vi "Find PID in Configuration.vi"(10 "Channels":T1={"ID"="", "Setpoint"=refnum, "Process Variable"=refnum, "Output"=refnum, "PID gains"={"proportional gain (Kc)"=1.0, "integral time (Ti, min)"=0.01, "derivative time (Td, min)"=0.0}, "output range"={"output high"=100.0, "output low"=-100.0}} {"output range"."output low" format="%.2f"; "output range"."output high" format="%.2f"}, 11 "Tagbus PID Module configuration in":refnum<class "Tagbus PID Module configuration.lvclass">) -> (2 "index":i32, 3 "Tagbus PID Module configuration out":refnum<class "Tagbus PID Module configuration.lvclass">)   [LabVIEW 2014, in "Tagbus PID Module configuration.lvclass"]
doc: "This VI locates a given PID Loop in the Module Configuration and returns it's index if found, or -1 if not found."
uses:
  Tagbus PID Module configuration.lvclass
  <vilib>/NI/Tag Bus Module Framework/channel/TBM channel.lvclass
  Tagbus PID Module configuration.lvclass/Tagbus PID Module configuration.ctl
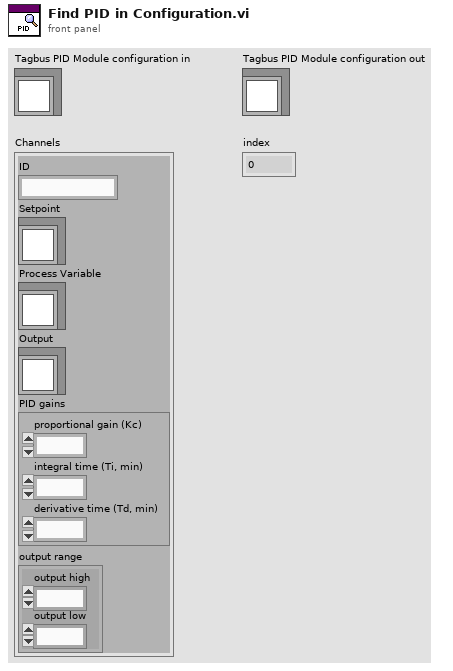
[diagram p1: front panel]
types:
  T1 = cluster{"ID":string, "Setpoint":refnum<class "TBM channel.lvclass">, "Process Variable":refnum<class "TBM channel.lvclass">, "Output":refnum<class "TBM channel.lvclass">, "PID gains":cluster{"proportional gain (Kc)":dbl, "integral time (Ti, min)":dbl, "derivative time (Td, min)":dbl}, "output range":cluster{"output high":dbl, "output low":dbl}}
  T2 = cluster{"ID":string, "Setpoint":refnum<class "TBM channel.lvclass">, "Process Variable":refnum<class "TBM channel.lvclass">, "Output":refnum<class "TBM channel.lvclass">, "PID gains":cluster{"proportional gain (Kc)":dbl, "integral time (Ti, min)":dbl, "derivative time (Td, min)":dbl}, "output range":cluster{"output high":dbl, "output low":dbl}}[]
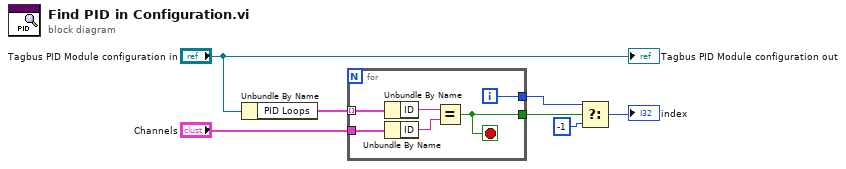
[diagram p0: block diagram]
diagram:
  n1 = Unbundle By Name("Tagbus PID Module configuration in") -> ("PID Loops"=w2:T2)
  n2 = for {
    tunnel: "Channels" -> [w13]
    tunnel: [w10] -> w4
    tunnel: [w9] -> w5
    tunnel: w2 -> [w8] mode=indexing
    i -> [w10]
    stop <- w9 stop-if-true
    n3 = Unbundle By Name(w8) -> ("ID"=w11:string)
    n4 = Unbundle By Name(w13) -> ("ID"=w12:string)
    n5 = Equal?(x=w11, y=w12) -> (x = y?=w9:bool)
  }
  n6 = Select(t=w4, s=w5, f=-1) -> (s? t:f=→"index":i32)
  "Tagbus PID Module configuration out" <- "Tagbus PID Module configuration in"
